vi "Tx Inline Start.vi"(8 "error in (no error)":errorcluster, 11 "Framework in":refnum<class "Framework.lvclass">) -> (0 "error out":errorcluster, 3 "Framework out":refnum<class "Framework.lvclass">)   [LabVIEW 2017, in "DSF Core.lvlib" / "Framework.lvclass"]
uses:
  Framework.lvclass
  Framework.lvclass/Framework.ctl
  Plugin/Plugin.lvclass
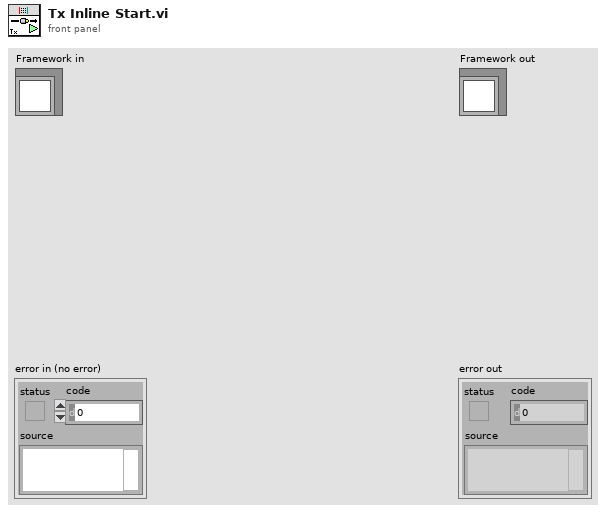
[diagram p1: front panel]
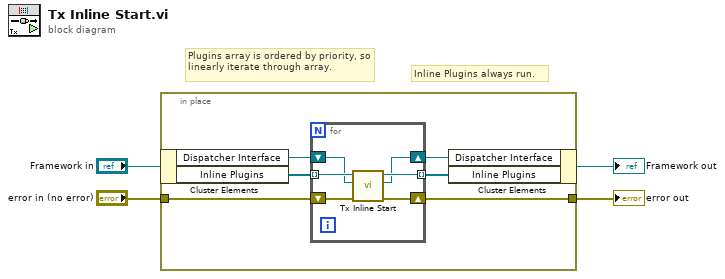
[diagram p0: block diagram]
diagram:
  # "Inline Plugins always run."
  # "Plugins array is ordered by priority, so linearly iterate through array."
  n1 = in-place {
    in-place-border: "error in (no error)" -> [w10]
    in-place-border: [w9] -> w3
    n2 = in-place-cluster #1("Framework in") -> ("Dispatcher Interface"=w6:refnum<class "Dispatcher Interface.lvclass">, "Inline Plugins"=w8:refnum<class "Plugin.lvclass">[])
    n3 = for {
      tunnel: w8 -> [w12] mode=indexing
      tunnel: [w16] -> w7 mode=indexing
      shift-right: [w15] -> w9
      shift-left: w10 -> [w14]
      shift-right: [w13] -> w5
      shift-left: w6 -> [w11]
      n4 = call "Tx Inline Start.vi"("error in (no error)"=w14, "Dispatcher Interface in"=w11, "Plugin in"=w12) -> ("error out"=w15:errorcluster, "Dispatcher Interface out"=w13:refnum<class "Dispatcher Interface.lvclass">, "Plugin out"=w16:refnum<class "Plugin.lvclass">)  [unwired: 6 in]
    }
    n5 = in-place-cluster #1("Dispatcher Interface"=w5, "Inline Plugins"=w7) -> (→"Framework out":refnum<class "Framework.lvclass">)
  }
  "error out" <- w3
